vi "JL_Button_Press.vi"(0 "GEA2 Reference In":refnum<k24>, 5 "GEA Inputs":T1={"Source"=228, "Destination"=36} {"Destination" format="%.0x"; "Source" format="%.0x"}, 9 "Button":T2, 11 "Error In":errorcluster, 12 "Hold Time (s)":dbl=0.5 format="%#_13g") -> (4 "GEA2 Reference Out":refnum<k24>, 15 "Error Out":errorcluster)   [LabVIEW 2016]
uses:
  Q:/Common/DLLs/GEA3/GeaCommunication.dll
  Common/DLLs/GEA3/GeaCommunication.dll
  Type Defs/JL_Buttons.ctl
  Common/LabVIEW GEA2 Toolkit/LabVIEW_GEA2_Toolkit.lvlibp/type defs/Source_Destination.ctl
  Common/LabVIEW GEA2 Toolkit/LabVIEW_GEA2_Toolkit.lvlibp/type defs/ERD Write Data In.ctl
  Common/LabVIEW GEA2 Toolkit/LabVIEW_GEA2_Toolkit.lvlibp/type defs/Data Type.ctl
  <vilib>/DAQmx/write.llb/DAQmx Write (Digital 1D Bool NChan 1Samp 1Line).vi
  <vilib>/DAQmx/write.llb/DAQmx Write (Digital Bool 1Line 1Point).vi
  <vilib>/DAQmx/create/channels.llb/DAQmx Create Channel (DO-Digital Output).vi
  <vilib>/DAQmx/miscellaneous.llb/DAQmx Fill In Error Info.vi
  Common/LabVIEW GEA2 Toolkit/LabVIEW_GEA2_Toolkit.lvlibp
panel:
  out "SLB?":bool
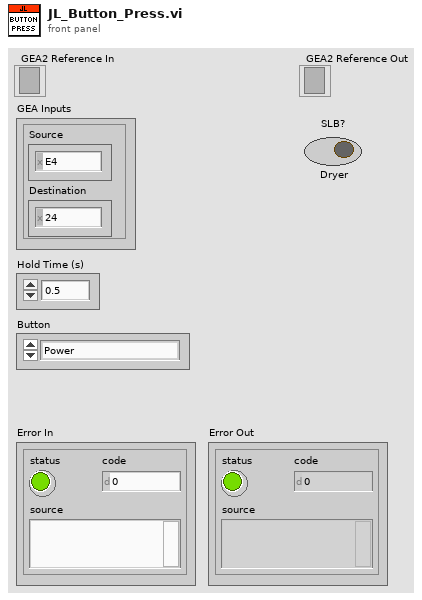
[diagram p1: front panel]
types:
  T1 = typedef "LabVIEW_GEA2_Toolkit.lvlibp/Source_Destination.ctl" = cluster{"Source":u8, "Destination":u8}
  T2 = typedef "JL_Buttons.ctl" = enum16{"Power", "Start / Pause ", "Temp Option ", "Dryness Level", "Time Option", "Time Increment ", "Time Decrement ", "MyCycle", "eDry ", "Delay", "Extended Tumble", "Control Lock", "Volume/Signal", "Damp Alert / Drum Light", "Unused", "(SW213)", "(SW322)", "Clear / Reset"}
  T3 = typedef "LabVIEW_GEA2_Toolkit.lvlibp/ERD Write Data In.ctl" = cluster{"ERD Number":u16, "Data Type":T4, "Data":string}
  T4 = typedef "LabVIEW_GEA2_Toolkit.lvlibp/Data Type.ctl" = enum16{"string", "boolean", "uint8_t", "uint16_t", "uint32_t", "uint64_t", "int8_t", "int16_t", "int32_t", "int64_t"}
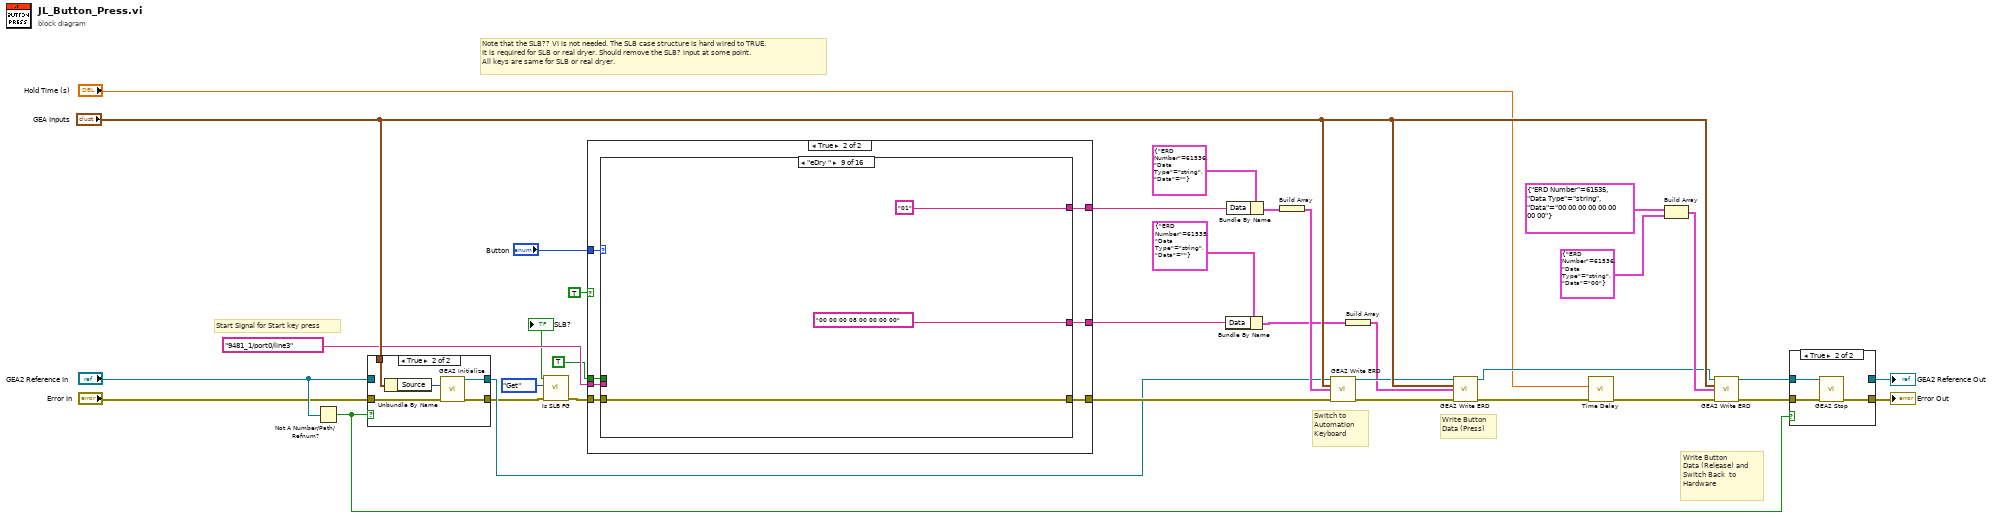
[diagram p0: block diagram]
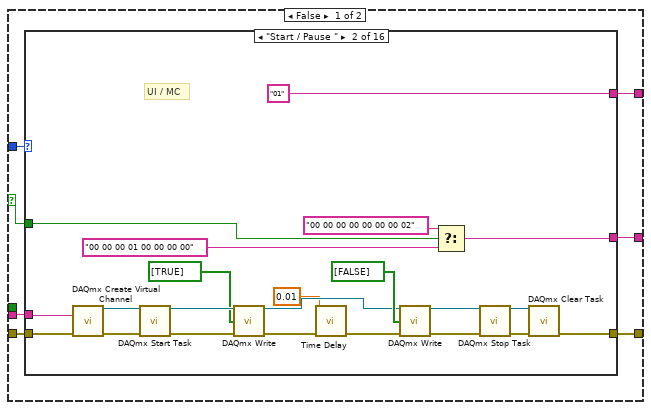
[diagram p2: hidden frame]
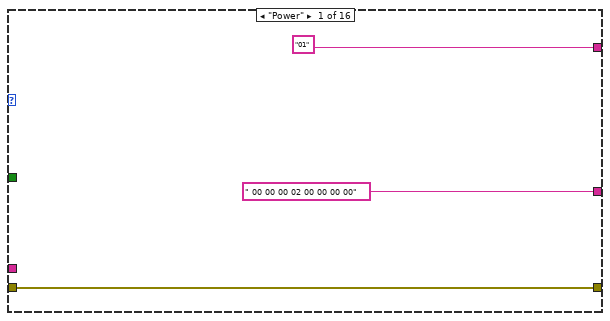
[diagram p3: hidden frame]
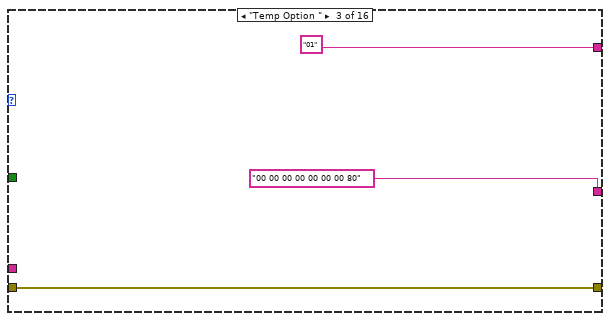
[diagram p4: hidden frame]
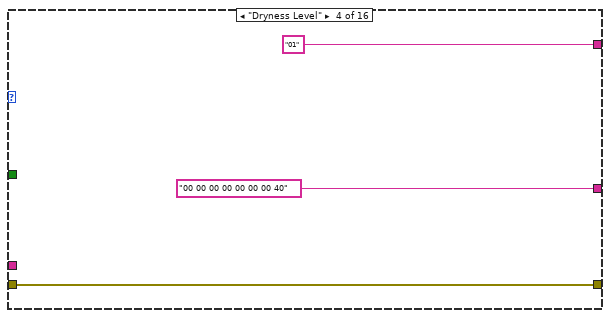
[diagram p5: hidden frame]
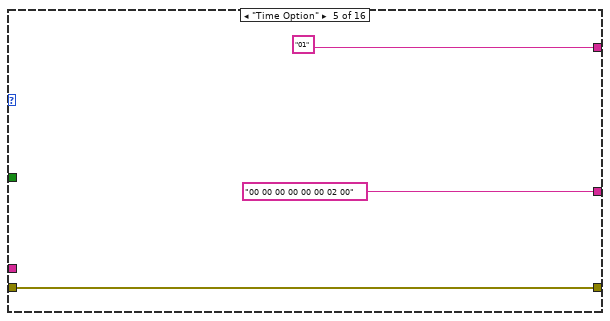
[diagram p6: hidden frame]
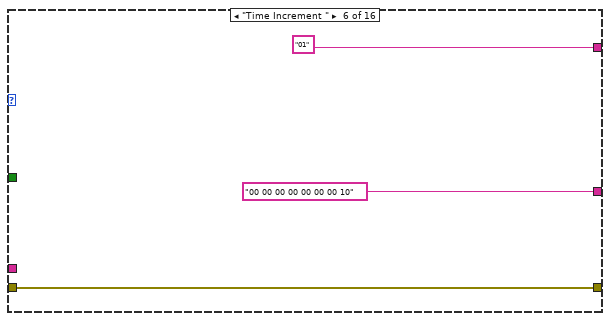
[diagram p7: hidden frame]
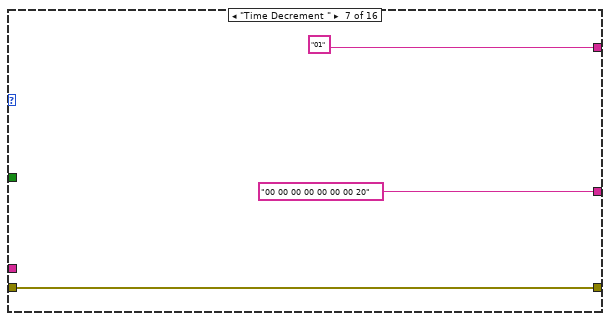
[diagram p8: hidden frame]
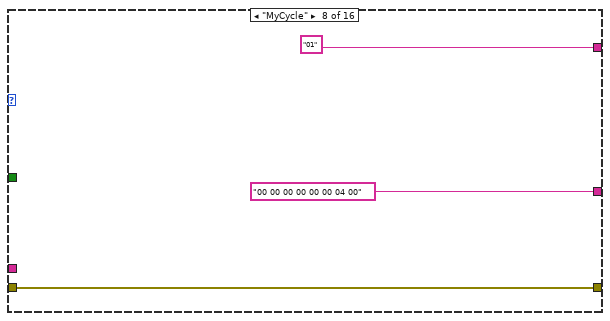
[diagram p9: hidden frame]
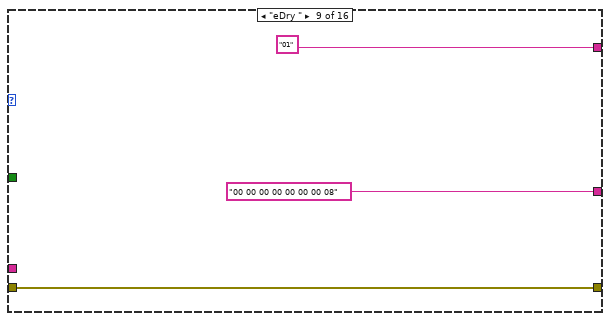
[diagram p10: hidden frame]
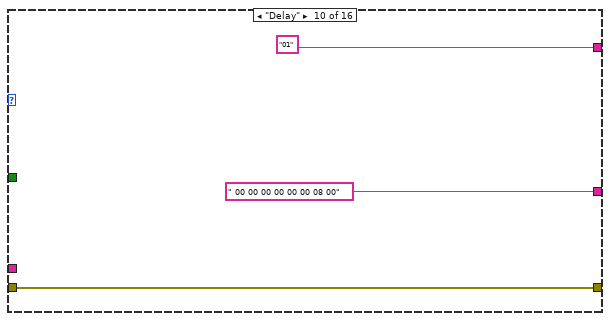
[diagram p11: hidden frame]
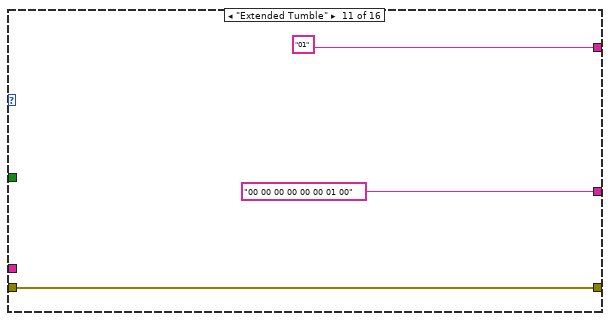
[diagram p12: hidden frame]
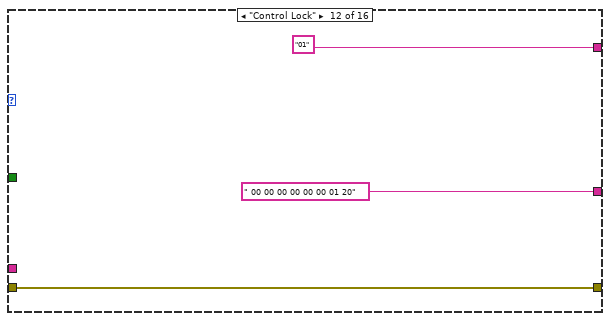
[diagram p13: hidden frame]
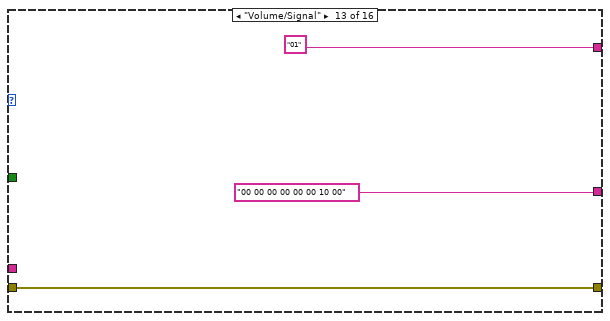
[diagram p14: hidden frame]
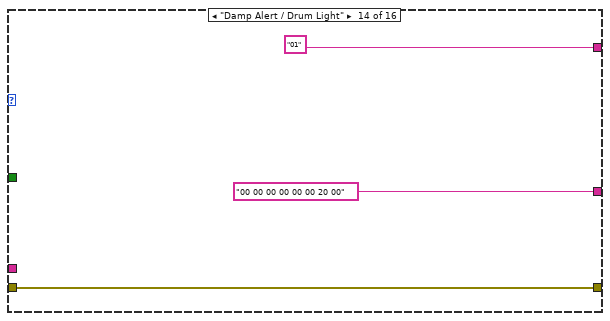
[diagram p15: hidden frame]
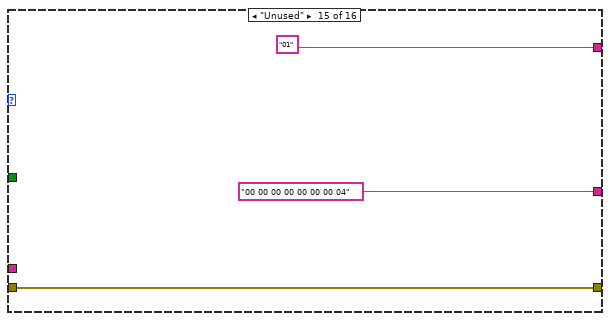
[diagram p16: hidden frame]
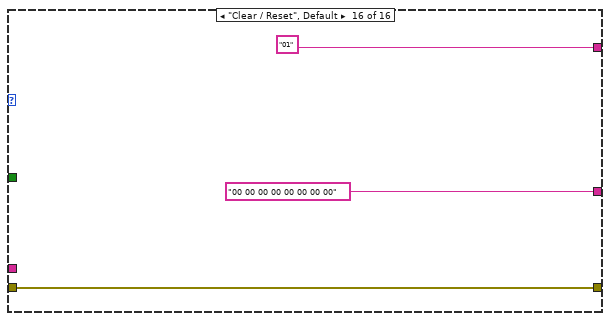
[diagram p17: hidden frame]
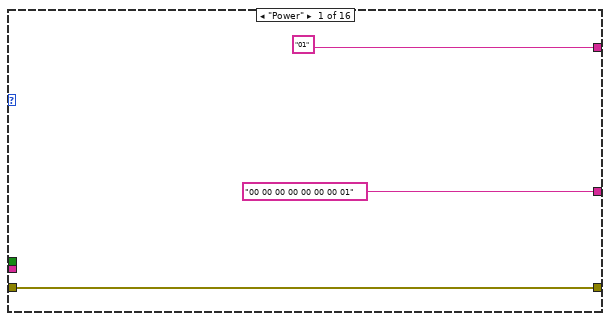
[diagram p18: hidden frame]
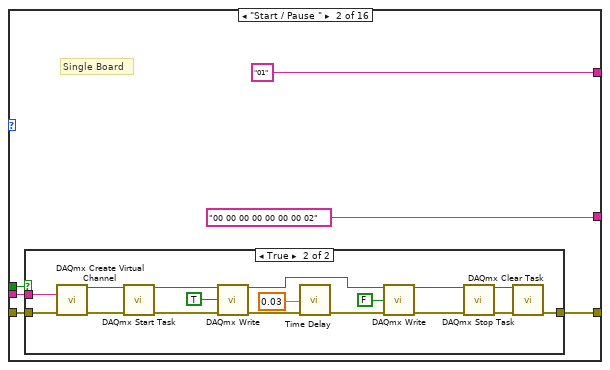
[diagram p19: hidden frame]
diagram:
  # "Note that the SLB?? VI is not needed. The SLB case structure is hard wired to TRUE.\nIt is required for SLB or real dryer. Should remove the SLB? input at some point.\nAll keys are same for SLB or real dryer."
  # "Start Signal for Start key press"
  # "Write Button\nData (Release) and \nSwitch Back  to\nHardware"
  # "Write Button\nData (Press)"
  # "Switch to\nAutomation \nKeyboard"
  n1 = Not A Number/Path/Refnum?(number/path/refnum="GEA2 Reference In") -> (NaN/Path/Refnum?=w32:bool)
  n2 = case shown="True" w32 {
    tunnel: "Error In" -> [w36 w42]
    tunnel: [w36 w41] -> w5
    tunnel: "GEA2 Reference In" -> [w37 _]
    tunnel: [w37 w40] -> w7
    tunnel: "GEA Inputs" -> [_ w38]
    frame False {
    }
    frame True {
      n3 = Unbundle By Name(w38) -> ("Source"=w39:u8)
      n4 = call "GEA2 Initialize.vi"("Source Address"=w39, "error in"=w42) -> ("GEA2 Reference Out"=w40:refnum<k24>, "error out"=w41:errorcluster)  [unwired: 11 in, 1 out]
    }
  }
  n5 = call "Is SLB FG.vi"("Error In"=w5, "Action"=enum16{"Get", "Set"}."Get") -> ("Error Out"=w4:errorcluster, "SLB"=→"SLB?":bool)  [unwired: 8 in]
  n6 = case shown="True" TRUE {
    selector: TRUE -> [w43 _]
    tunnel: [w45 w123] -> w14
    tunnel: [w46 w122] -> w13
    tunnel: w4 -> [w48 w121]
    tunnel: tag "9481_1/port0/line3" ("Line(s)") -> [w49 w120]
    tunnel: "Button" -> [w44 w119]
    tunnel: [w47 w118] -> w8
    tunnel: TRUE ("SLB") -> [_ w117]
    frame False {
      n7 = case shown="\"Start / Pause \"" w44 {
        tunnel: ["01" "01" "01" "01" "01" "01" "01" "01" "01" "01" "01" "01" "01" "01" "01" "01"] -> w45
        tunnel: [" 00 00 00 02 00 00 00 00" w53 "00 00 00 00 00 00 00 80" "00 00 00 00 00 00 00 40" "00 00 00 00 00 00 02 00" "00 00 00 00 00 00 00 10" "00 00 00 00 00 00 00 20" "00 00 00 00 00 00 04 00" "00 00 00 00 00 00 00 08" " 00 00 00 00 00 00 08 00" "00 00 00 00 00 00 01 00" " 00 00 00 00 00 00 01 20" "00 00 00 00 00 00 10 00" "00 00 00 00 00 00 20 00" "00 00 00 00 00 00 00 04" "00 00 00 00 00 00 00 00"] -> w46
        tunnel: w49 -> [_ w67 _ _ _ _ _ _ _ _ _ _ _ _ _ _]
        tunnel: [w50 w64 w75 w78 w81 w84 w87 w90 w93 w96 w99 w102 w105 w108 w111 w114] -> w47
        tunnel: w48 -> [w50 w58 w75 w78 w81 w84 w87 w90 w93 w96 w99 w102 w105 w108 w111 w114]
        tunnel: w43 -> [_ w54 _ _ _ _ _ _ _ _ _ _ _ _ _ _]
        frame "Power" {
        }
        frame "Start / Pause " {
          # "UI / MC"
          n8 = call-poly <vilib>:"DAQmx Create Virtual Channel.vi"("lines"=w67, "error in"=w58) -> ("task out"=w70:refnum<k21>, "error out"=w71:errorcluster)  [unwired: 12 in]
          n9 = call <vilib>:"DAQmx Start Task.vi"("task/channels in"=w70, "error in"=w71) -> ("task out"=w73:refnum<k21>, "error out"=w72:errorcluster)  [unwired: 12 in]
          n10 = call-poly <vilib>:"DAQmx Write.vi"("task/channels in"=w73, "data"=bool[] [TRUE], "error in"=w72) -> ("task out"=w59:refnum<k21>, "error out"=w61:errorcluster)  [unwired: 10 in, 1 out]
          n11 = call "Time Delay"("error in (no error)"=w61, "Delay Time (s)"=0.01) -> ("error out"=w60:errorcluster)  [unwired: 9 in]
          n12 = call-poly <vilib>:"DAQmx Write.vi"("task/channels in"=w59, "data"=bool[] [FALSE], "error in"=w60) -> ("task out"=w66:refnum<k21>, "error out"=w65:errorcluster)  [unwired: 10 in, 1 out]
          n13 = Select(t="00 00 00 00 00 00 00 02", s=w54, f="00 00 00 01 00 00 00 00") -> (s? t:f=w53:string)
          n14 = call <vilib>:"DAQmx Stop Task.vi"("task/channels in"=w66, "error in"=w65) -> ("task out"=w69:refnum<k21>, "error out"=w68:errorcluster)  [unwired: 12 in]
          n15 = call <vilib>:"DAQmx Clear Task.vi"("task in"=w69, "error in"=w68) -> ("error out"=w64:errorcluster)  [unwired: 13 in]
        }
        frame "Temp Option " {
        }
        frame "Dryness Level" {
        }
        frame "Time Option" {
        }
        frame "Time Increment " {
        }
        frame "Time Decrement " {
        }
        frame "MyCycle" {
        }
        frame "eDry " {
        }
        frame "Delay" {
        }
        frame "Extended Tumble" {
        }
        frame "Control Lock" {
        }
        frame "Volume/Signal" {
        }
        frame "Damp Alert / Drum Light" {
        }
        frame "Unused" {
        }
        frame "Clear / Reset", Default {
        }
      }
    }
    frame True {
      n16 = case shown="\"eDry \"" w119 {
        tunnel: ["01" "01" "01" "01" "01" "01" "01" "01" "01" "01" "01" "01" "01" "01" "01" "01"] -> w123
        tunnel: ["00 00 00 00 00 00 00 01" "00 00 00 00 00 00 00 02" "00 00 00 80 00 00 00 00" "00 00 00 40 00 00 00 00" "00 00 02 00 00 00 00 00" "00 00 00 10 00 00 00 00" "00 00 00 20 00 00 00 00" "00 00 04 00 00 00 00 00" "00 00 00 08 00 00 00 00" "00 00 08 00 00 00 00 00" "00 00 01 00 00 00 00 00" "00 00 01 20 00 00 00 00" "00 00 10 00 00 00 00 00" "00 00 20 00 00 00 00 00" "00 00 00 00 00 00 00 04" "00 00 00 00 00 00 00 00"] -> w122
        tunnel: w120 -> [_ w130 _ _ _ _ _ _ _ _ _ _ _ _ _ _]
        tunnel: [w124 w129 w151 w154 w157 w160 w163 w166 w169 w172 w175 w178 w181 w184 w187 w190] -> w118
        tunnel: w121 -> [w124 w128 w151 w154 w157 w160 w163 w166 w169 w172 w175 w178 w181 w184 w187 w190]
        tunnel: w117 -> [_ w127 _ _ _ _ _ _ _ _ _ _ _ _ _ _]
        frame "Power" {
        }
        frame "Start / Pause " {
          # "Single Board"
          n17 = case shown="True" w127 {
            tunnel: w130 -> [_ w144]
            tunnel: [w133 w141] -> w129
            tunnel: w128 -> [w133 w137]
            frame False {
            }
            frame True {
              n18 = call-poly <vilib>:"DAQmx Create Virtual Channel.vi"("lines"=w144, "error in"=w137) -> ("task out"=w147:refnum<k21>, "error out"=w148:errorcluster)  [unwired: 12 in]
              n19 = call <vilib>:"DAQmx Start Task.vi"("task/channels in"=w147, "error in"=w148) -> ("task out"=w150:refnum<k21>, "error out"=w149:errorcluster)  [unwired: 12 in]
              n20 = call-poly <vilib>:"DAQmx Write.vi"("task/channels in"=w150, "data"=TRUE ("Boolean"), "error in"=w149) -> ("task out"=w138:refnum<k21>, "error out"=w140:errorcluster)  [unwired: 10 in, 1 out]
              n21 = call "Time Delay"("error in (no error)"=w140, "Delay Time (s)"=0.03) -> ("error out"=w139:errorcluster)  [unwired: 9 in]
              n22 = call-poly <vilib>:"DAQmx Write.vi"("task/channels in"=w138, "data"=FALSE ("Boolean"), "error in"=w139) -> ("task out"=w143:refnum<k21>, "error out"=w142:errorcluster)  [unwired: 10 in, 1 out]
              n23 = call <vilib>:"DAQmx Stop Task.vi"("task/channels in"=w143, "error in"=w142) -> ("task out"=w146:refnum<k21>, "error out"=w145:errorcluster)  [unwired: 12 in]
              n24 = call <vilib>:"DAQmx Clear Task.vi"("task in"=w146, "error in"=w145) -> ("error out"=w141:errorcluster)  [unwired: 13 in]
            }
          }
        }
        frame "Temp Option " {
        }
        frame "Dryness Level" {
        }
        frame "Time Option" {
        }
        frame "Time Increment " {
        }
        frame "Time Decrement " {
        }
        frame "MyCycle" {
        }
        frame "eDry " {
        }
        frame "Delay" {
        }
        frame "Extended Tumble" {
        }
        frame "Control Lock" {
        }
        frame "Volume/Signal" {
        }
        frame "Damp Alert / Drum Light" {
        }
        frame "Unused" {
        }
        frame "Clear / Reset", Default {
        }
      }
    }
  }
  n25 = Bundle By Name(cluster=T3 {"ERD Number"=61535, "Data Type"=enum."string", "Data"=""} ("ERD Write Data In"), "Data"=w13) -> (w18:T3)
  n26 = Bundle By Name(cluster=T3 {"ERD Number"=61536, "Data Type"=enum."string", "Data"=""} ("ERD Write Data In"), "Data"=w14) -> (w29:T3)
  n27 = Build Array(w29) -> (w28:T3[])
  n28 = call "GEA2 Write ERD.vi"("GEA2 Reference In"=w7, "GEA Inputs"="GEA Inputs", "Write ERD List"=w28, "Error In"=w8) -> ("GEA2 Reference Out"=w20:refnum<k24>, "Error Out"=w23:errorcluster)  [unwired: 9 in, 1 out]
  n29 = Build Array(w18) -> (w17:T3[])
  n30 = call "GEA2 Write ERD.vi"("GEA2 Reference In"=w20, "GEA Inputs"="GEA Inputs", "Write ERD List"=w17, "Error In"=w23) -> ("GEA2 Reference Out"=w19:refnum<k24>, "Error Out"=w22:errorcluster)  [unwired: 9 in, 1 out]
  n31 = call "Time Delay"("error in (no error)"=w22, "Delay Time (s)"="Hold Time (s)") -> ("error out"=w26:errorcluster)  [unwired: 9 in]
  n32 = Build Array(T3 {"ERD Number"=61535, "Data Type"=enum."string", "Data"="00 00 00 00 00 00 00 00"} ("ERD Write Data In"), T3 {"ERD Number"=61536, "Data Type"=enum."string", "Data"="00"} ("ERD Write Data In")) -> (w27:T3[])
  n33 = call "GEA2 Write ERD.vi"("GEA2 Reference In"=w19, "GEA Inputs"="GEA Inputs", "Write ERD List"=w27, "Error In"=w26) -> ("GEA2 Reference Out"=w24:refnum<k24>, "Error Out"=w25:errorcluster)  [unwired: 9 in, 1 out]
  n34 = case shown="True" w32 {
    tunnel: [w193 w197] -> w35
    tunnel: w24 -> [w194 w196]
    tunnel: [w194 _] -> w34
    tunnel: w25 -> [w193 w195]
    frame False {
    }
    frame True {
      n35 = call "GEA2 Stop.vi"("GEA2 Reference In"=w196, "Error In"=w195) -> ("Error Out"=w197:errorcluster)  [unwired: 13 in]
    }
  }
  "Error Out" <- w35
  "GEA2 Reference Out" <- w34
